vi "Creat Update cmd.vi"(8 "error in (no error)":errorcluster, 9 "Data":string[](array[string]), 10 "columns":string[](array[string]), 11 "table name":string) -> (0 "error out":errorcluster, 3 "insert query":string)   [LabVIEW 2014]
uses:
  <vilib>/addons/database/NI_Database_API.lvlib
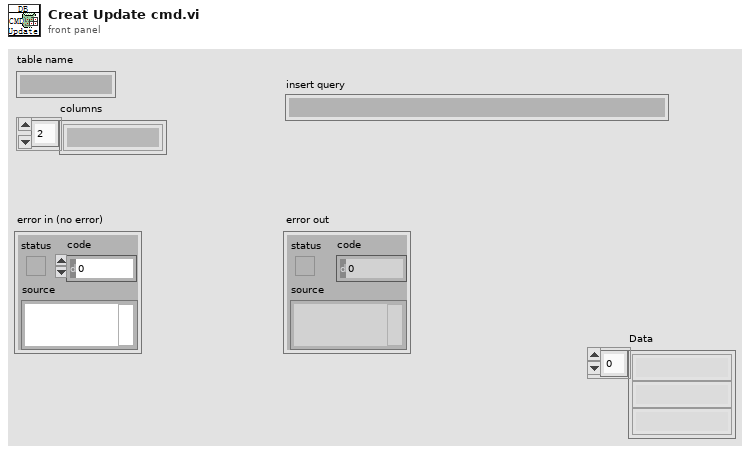
[diagram p1: front panel]
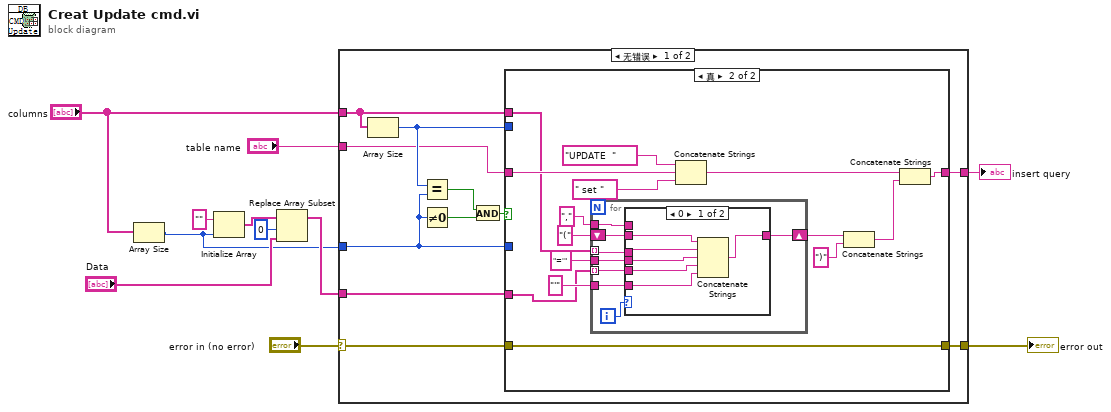
[diagram p0: block diagram]
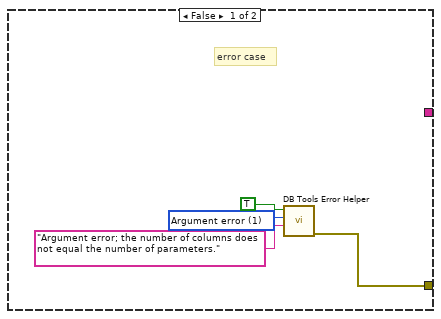
[diagram p2: hidden frame]
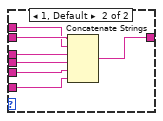
[diagram p3: hidden frame]
diagram:
  n1 = Array Size(array="columns") -> (size(s)=w1:i32)
  n2 = Initialize Array("", w1) -> (w6:string[])
  n3 = Replace Array Subset(array=w6, new element="Data", index=0 ("索引")) -> (w3:string[])
  n4 = case shown="无错误" "error in (no error)" {
    selector: "error in (no error)" -> [w19 w63]
    tunnel: [w18 w63] -> w10
    tunnel: "columns" -> [w17 _]
    tunnel: w1 -> [w16 _]
    tunnel: [w15 _] -> w9
    tunnel: "table name" -> [w14 _]
    tunnel: w3 -> [w13 _]
    frame No Error {
      n5 = Array Size(array=w17) -> (size(s)=w20:i32)
      n6 = Equal?(x=w20, y=w16) -> (x = y?=w12:bool)
      n7 = Not Equal To 0?(x=w16) -> (x != 0?=w22:bool)
      n8 = And(x=w12, y=w22) -> (x .and. y?=w21:bool)
      n9 = case shown="真" w21 {
        tunnel: w17 -> [_ w35]
        tunnel: w20 -> [_ _]
        tunnel: w16 -> [_ _]
        tunnel: w19 -> [_ w40]
        tunnel: [w26 w40] -> w18
        tunnel: [_ w39] -> w15
        tunnel: w14 -> [_ w38]
        tunnel: w13 -> [_ w28]
        frame False {
          w24 = 1 items=["No error", "Argument error", "Memory is full", "Out of zone", "End of file", "File already open", "Generic file I/O error", "File not found", "File permission error", "Disk is full", "Duplicate path", "Too many files open", "System feature not enabled", "Resource file not found", "Cannot add resource", "Resource not found", "Image not found", "Image memory error", "Pen does not exist", "Config type invalid", "Config token not found", "Config parse error", "Config memory error", "Bad external code format", "Bad external code offset", "External code not present", "Null window", "Destroy window error", "Null menu", "Print aborted", "Bad print record", "Print driver error", "Windows error during printing", "Memory error during printing", "Print dialog error", "Generic print error", "Invalid device refnum", "Device not found", "Device parameter error", "Device unit error", "Cannot open device", "Device call aborted", "Generic error", "Cancelled by user", "Object ID too low", "Object ID too high", "Object not in heap", "Unknown heap", "Unknown object (invalid DefProc)", "Unknown object (DefProc not in table)", "Message out of range", "Invalid (null) method", "Unknown message", "Manager call not supported", "Bad address", "Network operation in progress", "Network operation timed out", "Connection is busy", "Network attribute not supported", "Network error", "Address in use", "System out of memory", "Connection aborted", "Connection refused", "Not connected", "Already connected", "Connection closed", "Initialization error (interapplication manager)", "Bad occurrence", "Wait on unbound occurrence handler", "Occurrence queue overflow", "Datalog type conflict", "Unused", "Unrecognized type (interapplication manager)", "Memory corrupt", "Failed to make temporary DLL", "Old CIN version", "Drag socket not found", "Failed to load drop-object", "Failed to register OLE object", "Failed to release OLE object", "Format specifier type mismatch", "Unknown format specifier", "Too few format specifiers", "Too many format specifiers", "Scan failed", "Newer CIN version", "Error converting to variant", "Runtime menu error", "Password tampered", "Variant attribute not found", "Incompatible variant data type", "Event data is not available", "Event Store is not present", "Occurrence is not found", "Event Queue is not created", "Event info is not available", "Refnum passed is NULL", "Error retrieving Class GUID", "Error retrieving CoClass GUID", "Error retrieving TypeLib GUID.", "Bad built application magic bytes.", "Specific driver is different from the specific driver associated with the Logical Name.", "There is no session opened to the class driver.", "Max Error", "MAX - Error with config objects", "MAX - Error loading configuration", "MAX - Group not supported"]
          # "error case"
          n10 = call <vilib>:"DB Tools Error Helper.vi"("source"="Argument error; the number of columns does not equal the number of parameters.", "code"=w24, "status"=TRUE) -> ("error out"=w26:errorcluster)  [unwired: 1 in, 7 out]
        }
        frame True {
          n11 = for {
            tunnel: w35 -> [w49] mode=indexing
            tunnel: "='" -> [w48]
            tunnel: "'" -> [w45]
            shift-right: [w47] -> w31
            shift-left: "(" -> [w46]
            tunnel: w28 -> [w44] mode=indexing
            tunnel: "," -> [w42]
            i -> [w43]
            n12 = case shown="0" w43 {
              tunnel: w49 -> [w53 w62]
              tunnel: w48 -> [w52 w61]
              tunnel: [w54 w60] -> w47
              tunnel: w46 -> [w55 w57]
              tunnel: w45 -> [w50 w59]
              tunnel: w44 -> [w51 w58]
              tunnel: w42 -> [_ w56]
              frame 0 {
                n13 = Concatenate Strings(w55, w53, w52, w51, w50) -> (w54:string)
              }
              frame 1, Default {
                n14 = Concatenate Strings(w57, w56, w62, w61, w58, w59) -> (w60:string)
              }
            }
          }
          n15 = Concatenate Strings("UPDATE  " ("Substring"), w38, " set " ("Substring")) -> (w37:string)
          n16 = Concatenate Strings(w31, ")" ("字符串")) -> (w30:string)
          n17 = Concatenate Strings(w37, w30) -> (w39:string)
        }
      }
    }
    frame Error {
    }
  }
  "error out" <- w10
  "insert query" <- w9
